vi "Setup Temperature.vi"(0 "reference in":refnum<class "Temp.lvclass">, 3 "Module Names (NI-MAX Alias)":string[](array[string])=["Thermo-4CH"], 4 "Number of Channels Per Module":u32[](array[numeric])=[4], 5 "error in (no error)":errorcluster, 9 "Thermocouple Type":i32(ring)=10072 items=["J"=10072, "K"=10073, "N"=10077, "R"=10082, "S"=10085, "T"=10086, "B"=10047, "E"=10055], 11 "Temperature Units":i32(ring)=10144 items=["Deg C"=10143, "Deg F"=10144, "Kelvins"=10325, "Deg R"=10145, "From Custom Scale"=10065]) -> (14 "reference out":refnum<class "Temp.lvclass">, 19 "error out":errorcluster)   [LabVIEW 2017, in "Temp.lvclass"]
uses:
  Temp.lvclass
  <vilib>/DAQmx/create/channels.llb/DAQmx Create Channel (AI-Temperature-Thermocouple).vi
  <vilib>/DAQmx/configure/timing.llb/DAQmx Timing (Sample Clock).vi
  <resource>/objmgr/daqmx.rc
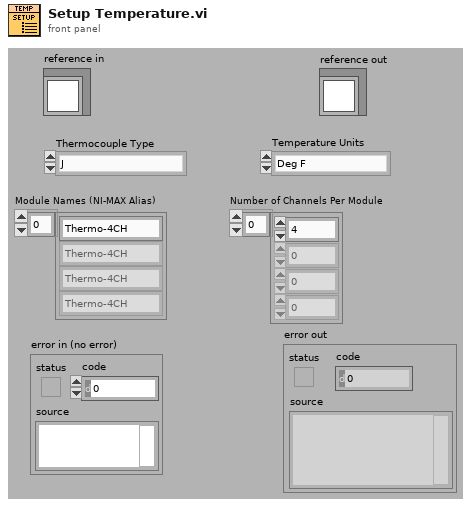
[diagram p1: front panel]
types:
  T1 = typedef "Temp.lvclass/ObjectAttributes.ctl" = cluster{"Temperature Task":refnum<k21>, "Temperature Readings":dbl[], "Thermocouple Type":i32, "Temperature Units":i32, "Average Temperature":dbl, "Number of Temperature Modules":i32, "Number of Total Temperature Channels":i32, "Temperature On/Off Status":bool, "Temperature Module Names (NI-Max Name)":string[], "Number of Channels Per Temperature  Module":i32[], "Temperature VI Reference":refnum<vi>}
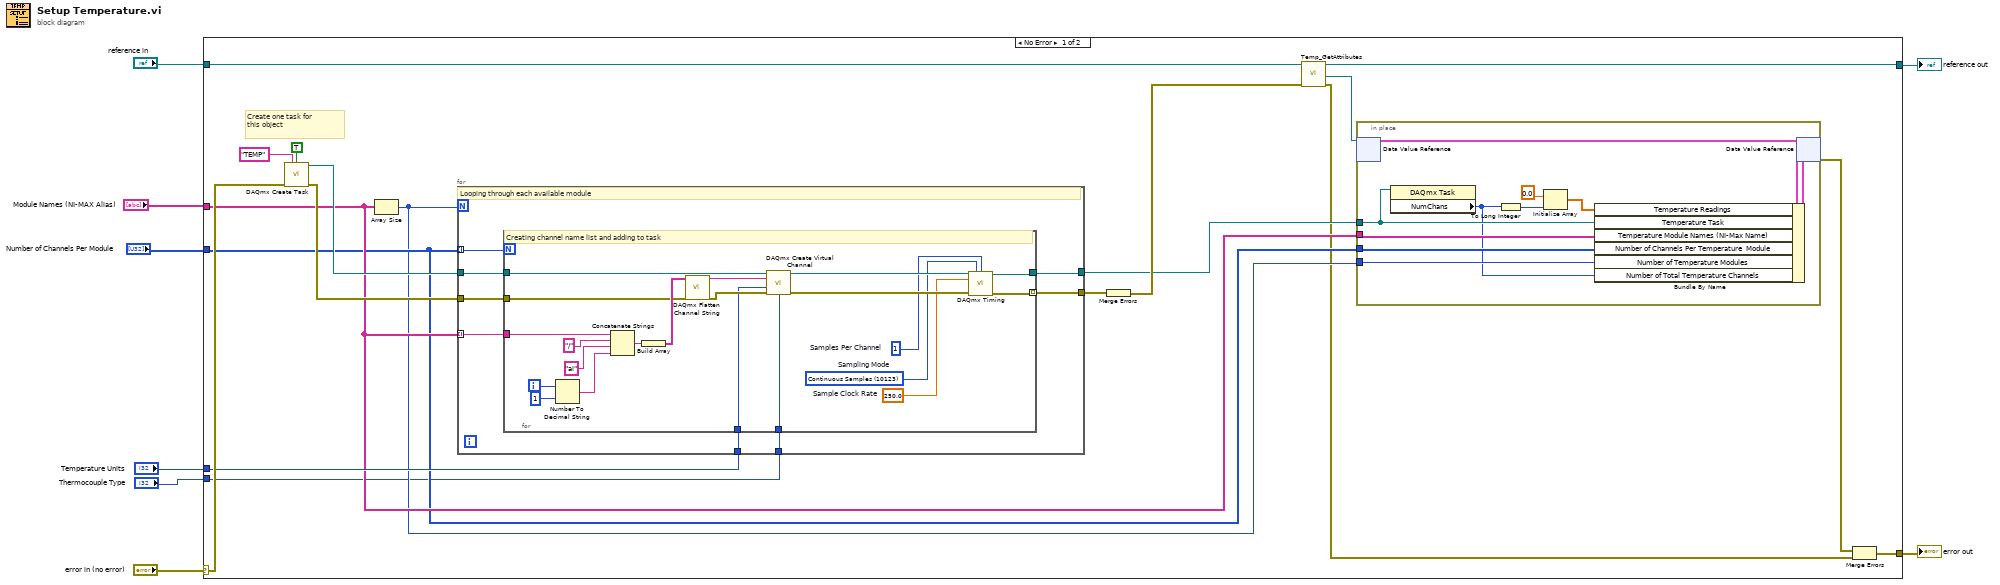
[diagram p0: block diagram]
diagram:
  n1 = case shown="No Error" "error in (no error)" {
    selector: "error in (no error)" -> [w17 w68]
    tunnel: [w24 w68] -> w7
    tunnel: [w25 w67] -> w5
    tunnel: "reference in" -> [w27 w67]
    tunnel: "Temperature Units" -> [w14 _]
    tunnel: "Module Names (NI-MAX Alias)" -> [w13 _]
    tunnel: "Number of Channels Per Module" -> [w12 _]
    tunnel: "Thermocouple Type" -> [w10 _]
    frame No Error {
      # "Create one task for \nthis object"
      n2 = call <vilib>:"DAQmx Create Task.vi"("new task name"="TEMP", "auto cleanup"=TRUE, "error in"=w17) -> ("task out"=w20:refnum<k21>, "error out"=w19:errorcluster)  [unwired: 11 in]
      n3 = Array Size(array=w13) -> (size(s)=w11:i32)
      n4 = for {
        N: w11 -> [_]
        tunnel: w12 -> [w35] mode=indexing
        tunnel: w20 -> [w34]
        tunnel: w19 -> [w33]
        tunnel: w13 -> [w32] mode=indexing
        tunnel: [w31] -> w18
        tunnel: [w30] -> w15
        tunnel: w14 -> [w29]
        tunnel: w10 -> [w28]
        # "Looping through each available module"
        n5 = for {
          N: w35 -> [_]
          tunnel: w34 -> [w50]
          tunnel: w33 -> [w47]
          tunnel: w32 -> [w46]
          tunnel: [w42] -> w30
          tunnel: [w40] -> w31 mode=indexing
          tunnel: w29 -> [w36]
          tunnel: w28 -> [w44]
          i -> [w56]
          w37 = 1  # Samples Per Channel
          w38 = 10123 items=["Finite Samples"=10178, "Continuous Samples"=10123, "Hardware Timed Single Point"=12522]  # Sampling Mode
          w39 = 250.0  # Sample Clock Rate
          # "Creating channel name list and adding to task"
          n6 = Number To Decimal String(number=w56, width (-)=i16 1) -> (decimal integer string=w53:string)
          n7 = Concatenate Strings(w46, "/", "ai", w53) -> (w49:string)
          n8 = Build Array(w49) -> (w48:string[])
          n9 = call <vilib>:"DAQmx Flatten Channel String.vi"("names in"=w48, "error in"=w47) -> ("names out"=w51:string, "error out"=w52:errorcluster)  [unwired: 12 in]
          n10 = call-poly <vilib>:"DAQmx Create Virtual Channel.vi"("task in"=w50, "physical channels"=w51, "units"=w36, "error in"=w52, "thermocouple type"=w44) -> ("task out"=w43:refnum<k21>, "error out"=w41:errorcluster)  [unwired: 9 in]
          n11 = call-poly <vilib>:"DAQmx Timing.vi"("task/channels in"=w43, "sample mode"=w38, "samples per channel"=w37, "rate"=w39, "error in"=w41) -> ("task out"=w42:refnum<k21>, "error out"=w40:errorcluster)  [unwired: 9 in]
        }
      }
      n12 = Merge Errors(w18) -> (w16:errorcluster)
      n13 = call "Temp_GetAttributes.vi"("reference in"=w27, "error in (no error)"=w16) -> ("reference out"=w25:refnum<class "Temp.lvclass">, "DataRef"=w23:refnum<data-value>, "error out"=w9:errorcluster)  [unwired: 14 in, 1 out]
      n14 = in-place {
        in-place-border: w15 -> [w64]
        in-place-border: w13 -> [w61]
        in-place-border: w12 -> [w60]
        in-place-border: w11 -> [w59]
        n15 = in-place-dvr #1(w23) -> (w65:T1)  [unwired: 1 out]
        n16 = property class="DAQmx Task"(reference=w64) -> ("NumChans"=w58:u32)  [unwired: 1 in, 2 out]
        n17 = To Long Integer(number=w58) -> (32bit integer=w57:i32)
        n18 = Initialize Array(0.0, w57) -> (w62:dbl[])
        n19 = Bundle By Name(cluster=w65, "Temperature Readings"=w62, "Temperature Task"=w64, "Temperature Module Names (NI-Max Name)"=w61, "Number of Channels Per Temperature  Module"=w60, "Number of Temperature Modules"=w59, "Number of Total Temperature Channels"=w58) -> (w66:T1)
        n20 = in-place-dvr #1(w66) -> (w26:errorcluster)  [unwired: 1 out]
      }
      n21 = Merge Errors(w26, w9) -> (w24:errorcluster)
    }
    frame Error {
    }
  }
  "error out" <- w7
  "reference out" <- w5
